vi "Contructor.vi"(8 "Error In":errorcluster, 9 "Speed [km/h]":dbl, 10 "ID":string, 11 "Spaceship in":refnum<class "Spaceship.lvclass">) -> (0 "Error Out":errorcluster, 3 "Spaceship out":refnum<class "Spaceship.lvclass">)   [LabVIEW 2021, in "Spaceship.lvclass"]
doc: "Init object of Spaceship class with all data and queue."
uses:
  Spaceship.lvclass
  Spaceship.lvclass/Spaceship.ctl
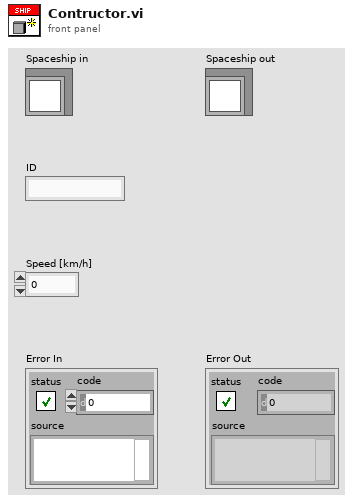
[diagram p1: front panel]
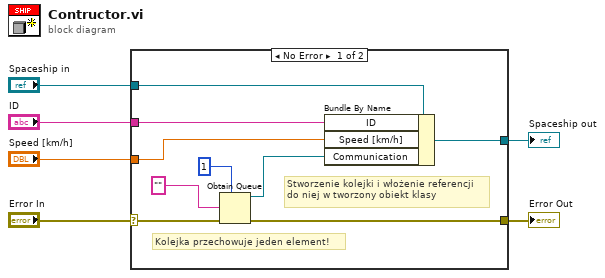
[diagram p0: block diagram]
diagram:
  n1 = case shown="No Error" "Error In" {
    selector: "Error In" -> [w8 w17]
    tunnel: [w7 w17] -> w5
    tunnel: [w14 w16] -> w3
    tunnel: "Spaceship in" -> [w15 w16]
    tunnel: "ID" -> [w13 _]
    tunnel: "Speed [km/h]" -> [w12 _]
    frame No Error {
      # "Kolejka przechowuje jeden element!"
      # "Stworzenie kolejki i włożenie referencji\ndo niej w tworzony obiekt klasy"
      n2 = Obtain Queue(max queue size (-1, unlimited)=1, element data type="", error in (no error)=w8) -> (queue out=w10:refnum<queue>, error out=w7:errorcluster)  [unwired: 2 in, 1 out]
      n3 = Bundle By Name(cluster=w15, "ID"=w13, "Speed [km/h]"=w12, "Communication"=w10) -> (w14:refnum<class "Spaceship.lvclass">)
    }
    frame Error {
    }
  }
  "Error Out" <- w5
  "Spaceship out" <- w3
